vi "Teleop.vi"(10 "Match Info":T1={"Autonomous Elapsed Seconds"=0.0, "TeleOp Elapsed Seconds"=0.0, "Disabled Elapsed Seconds"=0.0, "Visited Autonomous"=FALSE, "Visited TeleOp"=FALSE, "Visited Disabled"=FALSE, "Autonomous Settings"={"Autonomous Style"=enum."Independent", "VI Refnum"=refnum}}, 11 "Call Context":T2) -> ()   [LabVIEW 2013]
doc: "This VI is called for each TeleOp packet received from the DS where the robot is not disabled. It is often used to read from the joysticks and update I/O or to update setpoints for timed control loops. It should complete and return within 20 milliseconds or it may miss DS packets."
uses:
  <vilib>/Rock Robotics/WPI/DriverStation/WPI_DriverStationDerivedRobotMode.ctl
  <vilib>/Rock Robotics/WPI/DriverStation/WPI_DriverStationMatch Info.ctl
  Robot Global Data.vi
  <vilib>/Rock Robotics/WPI/Joystick/WPI_JoystickGetSetRefNum.vi
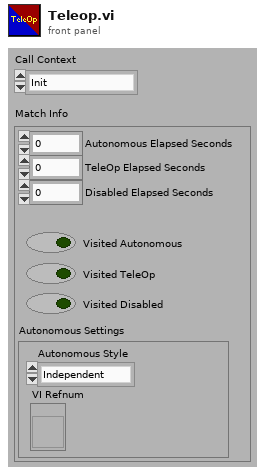
[diagram p1: front panel]
types:
  T1 = typedef "WPI_DriverStationMatch Info.ctl" = cluster{"Autonomous Elapsed Seconds":dbl, "TeleOp Elapsed Seconds":dbl, "Disabled Elapsed Seconds":dbl, "Visited Autonomous":bool, "Visited TeleOp":bool, "Visited Disabled":bool, "Autonomous Settings":cluster{"Autonomous Style":enum16{"Iterative", "Independent"}, "VI Refnum":refnum<vi>}}
  T2 = typedef "WPI_DriverStationDerivedRobotMode.ctl" = enum16{"Init", "Execute", "Stop"}
  T3 = typedef "WPI_JoystickDevRef.ctl" = cluster{"Device":T4}
  T4 = typedef "WPI_JoystickDeviceEnum.ctl" = enum16{"USB 1", "USB 2", "USB 3", "USB 4", "Kinect 1", "Kinect 2"}
  T5 = cluster{"axis 1 (x)":dbl, "axis 2 (y)":dbl, "axis 3 (throttle)":dbl, "axis 4":dbl, "axis 5":dbl, "axis 6":dbl}
  T6 = typedef "WPI_MotorControlDeviceRef.ctl" = cluster{"DeviceStatus":errorcluster, "Type":enum16{"PWM", "CAN"}, "PWM":cluster{"Digital Module":T7, "PWM Channel":T8, "DeadBand":T9}, "CAN":cluster{"Device Number":u8, "Control Mode":T10, "Semaphore":T11, "Max Vout":dbl}, "Invert":bool, "TransformRef":T12, "InvTransformRef":T12}
  T7 = typedef "FPGA_TypedefDigitalModule.ctl" = enum16{"Digital Module 1", "Digital Module 2"}
  T8 = typedef "FPGA_DIOPWMChannel.ctl" = enum8{"PWM 1", "PWM 2", "PWM 3", "PWM 4", "PWM 5", "PWM 6", "PWM 7", "PWM 8", "PWM 9", "PWM 10", "Invalid"}
  T9 = typedef "WPI_PWMDeadband.ctl" = cluster{"Name":string, "maxPositivePwm":i32, "minPositivePwm":i32, "centerPwm":i32, "maxNegativePwm":i32, "minNegativePwm":i32, "angularRange":u16}
  T10 = typedef "WPI_CANJaguar_ControlMode.ctl" = enum8{"Percent VBus", "Current", "Speed", "Position", "Voltage"}
  T11 = typedef "Semaphore RefNum" = refnum<k1>
  T12 = typedef "WPI_PWMTransform_ConPane.ctl" = refnum<vi>
  T13 = typedef "WPI_JoystickButtonState.ctl" = cluster{"Button 1":bool, "Button 2":bool, "Button 3":bool, "Button 4":bool, "Button 5":bool, "Button 6":bool, "Button 7":bool, "Button 8":bool, "Button 9":bool, "Button 10":bool, "Button 11":bool, "Button 12":bool}
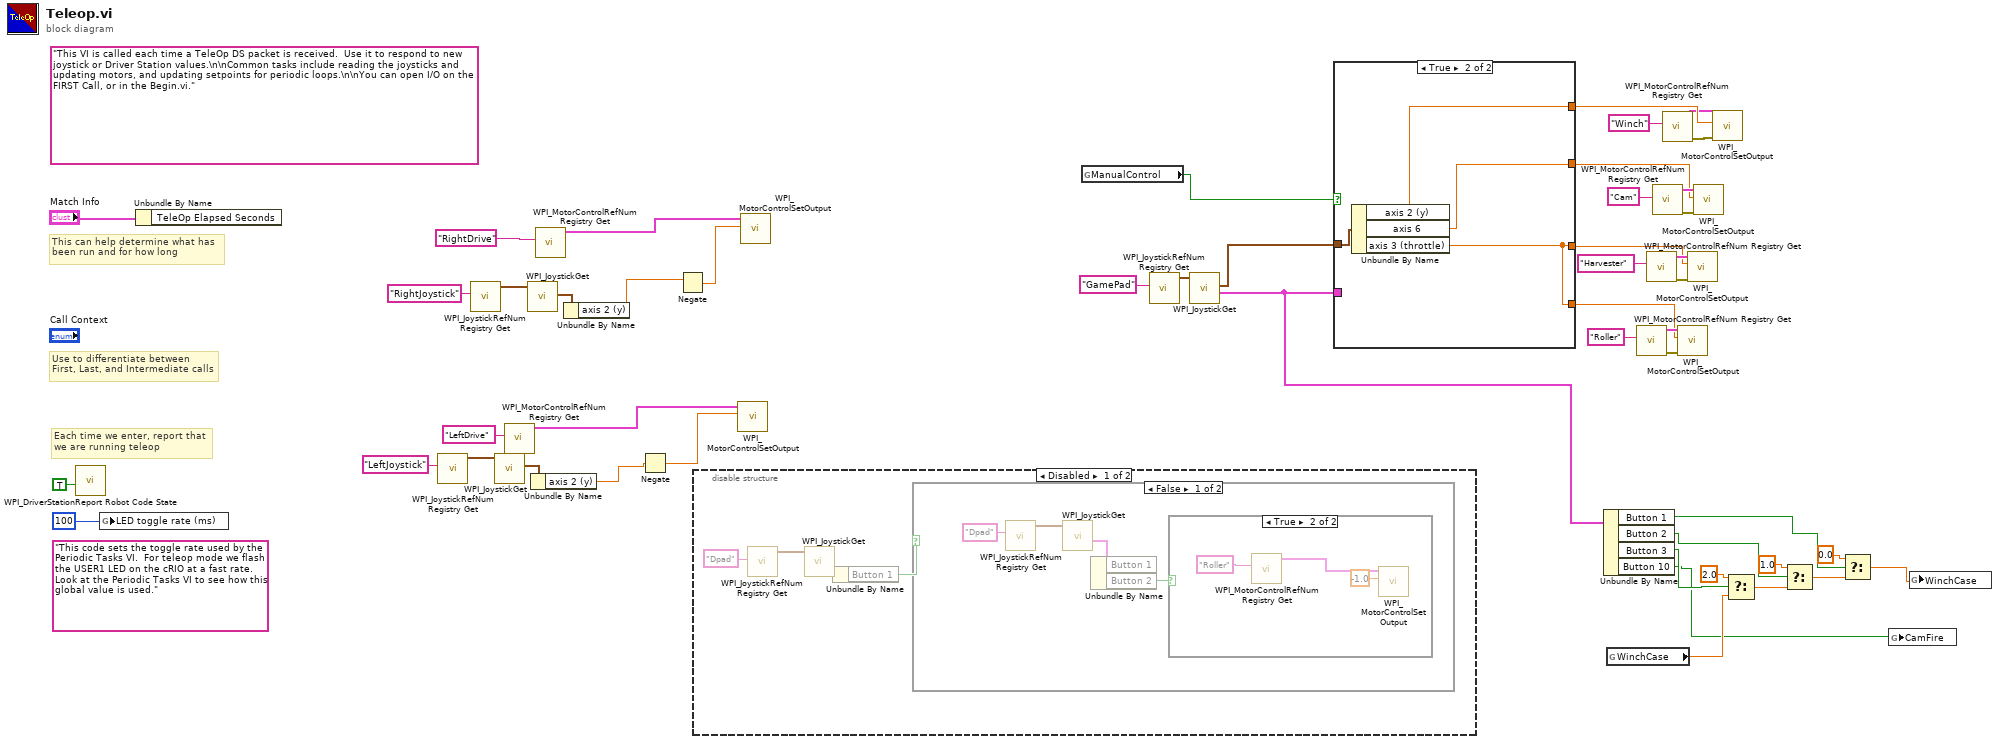
[diagram p0: block diagram]
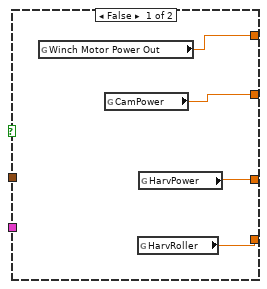
[diagram p2: hidden frame]
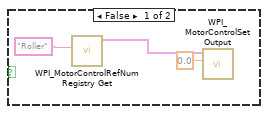
[diagram p3: hidden frame]
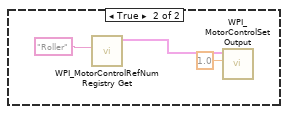
[diagram p4: hidden frame]
diagram:
  (unwired) "This code sets the toggle rate used by the Periodic Tasks VI.  For teleop mode we flash the USER1 LED on the cRIO at a fast rate.  Look at the Periodic Tasks VI to see how this global value is used."
  (unwired) "This VI is called each time a TeleOp DS packet is received.  Use it to respond to new joystick or Driver Station values.\n\nCommon tasks include reading the joysticks and updating motors, and updating setpoints for periodic loops.\n\nYou can open I/O on the FIRST Call, or in the Begin.vi."
  # "Each time we enter, report that\nwe are running teleop"
  # "Use to differentiate between\nFirst, Last, and Intermediate calls"
  # "This can help determine what has\nbeen run and for how long"
  n1 = call <vilib>:"WPI_DriverStationReport Robot Code State.vi"("TeleOp"=TRUE ("Autonomous")) -> ()  [unwired: 10 in, 1 out]
  n2 = global write "Robot Global Data.vi" "LED toggle rate (ms)"(u32 100 ("LED ms toggle rate")) -> ()
  n3 = Unbundle By Name("Match Info") -> ()  [unwired: 1 out]
  n4 = call <vilib>:"WPI_JoystickRefNum Registry Get.vi"("refnum name"="LeftJoystick") -> ("JoystickDevRef"=w38:T3)  [unwired: 9 in, 1 out]
  n5 = call <vilib>:"WPI_JoystickRefNum Registry Get.vi"("refnum name"="RightJoystick") -> ("JoystickDevRef"=w43:T3)  [unwired: 9 in, 1 out]
  n6 = call <vilib>:"WPI_JoystickGet.vi"("JoystickDevRef"=w38) -> ("Axes"=w37:T5)  [unwired: 4 in, 2 out]
  n7 = call <vilib>:"WPI_MotorControlRefNum Registry Get.vi"("refnum name"="LeftDrive") -> ("MotorControlDevRef"=w41:T6)  [unwired: 9 in, 1 out]
  n8 = call <vilib>:"WPI_JoystickGet.vi"("JoystickDevRef"=w43) -> ("Axes"=w42:T5)  [unwired: 4 in, 2 out]
  n9 = Unbundle By Name(w37) -> ("axis 2 (y)"=w36:dbl)
  n10 = call <vilib>:"WPI_MotorControlRefNum Registry Get.vi"("refnum name"="RightDrive") -> ("MotorControlDevRef"=w46:T6)  [unwired: 9 in, 1 out]
  n11 = Unbundle By Name(w42) -> ("axis 2 (y)"=w35:dbl)
  n12 = Negate(x=w36) -> (-x=w34:dbl)
  n13 = Negate(x=w35) -> (-x=w33:dbl)
  n14 = disable-structure shown="Disabled" {
    frame Disabled {
      n15 = call <vilib>:"WPI_JoystickRefNum Registry Get.vi"("refnum name"="Dpad") -> ("JoystickDevRef"=w52:T3)  [unwired: 9 in, 1 out]
      n16 = call <vilib>:"WPI_JoystickGet.vi"("JoystickDevRef"=w52) -> ("Buttons"=w51:T13)  [unwired: 4 in, 2 out]
      n17 = Unbundle By Name(w51) -> ("Button 1"=w50:bool)
      n18 = case shown="False" w50 {
        frame False {
          n19 = call <vilib>:"WPI_JoystickRefNum Registry Get.vi"("refnum name"="Dpad") -> ("JoystickDevRef"=w56:T3)  [unwired: 9 in, 1 out]
          n20 = call <vilib>:"WPI_JoystickGet.vi"("JoystickDevRef"=w56) -> ("Buttons"=w55:T13)  [unwired: 4 in, 2 out]
          n21 = Unbundle By Name(w55) -> ("Button 2"=w54:bool)  [unwired: 1 out]
          n22 = case shown="True" w54 {
            frame False {
              n23 = call <vilib>:"WPI_MotorControlRefNum Registry Get.vi"("refnum name"="Roller") -> ("MotorControlDevRef"=w59:T6)  [unwired: 9 in, 1 out]
              n24 = call <vilib>:"WPI_MotorControlSetOutput.vi"("Output"=0.0, "MotorControlDevRef"=w59) -> ()  [unwired: 7 in, 3 out]
            }
            frame True {
              n25 = call <vilib>:"WPI_MotorControlRefNum Registry Get.vi"("refnum name"="Roller") -> ("MotorControlDevRef"=w62:T6)  [unwired: 9 in, 1 out]
              n26 = call <vilib>:"WPI_MotorControlSetOutput.vi"("Output"=-1.0, "MotorControlDevRef"=w62) -> ()  [unwired: 7 in, 3 out]
            }
          }
        }
        frame True {
          n27 = call <vilib>:"WPI_MotorControlRefNum Registry Get.vi"("refnum name"="Roller") -> ("MotorControlDevRef"=w65:T6)  [unwired: 9 in, 1 out]
          n28 = call <vilib>:"WPI_MotorControlSetOutput.vi"("Output"=1.0, "MotorControlDevRef"=w65) -> ()  [unwired: 7 in, 3 out]
        }
      }
    }
    frame Enabled {
    }
  }
  n29 = call <vilib>:"WPI_MotorControlSetOutput.vi"("Output"=w34, "MotorControlDevRef"=w41) -> ()  [unwired: 7 in, 3 out]
  n30 = call <vilib>:"WPI_MotorControlSetOutput.vi"("Output"=w33, "MotorControlDevRef"=w46) -> ()  [unwired: 7 in, 3 out]
  n31 = global read "Robot Global Data.vi" "ManualControl"() -> (w21:bool)
  n32 = call <vilib>:"WPI_JoystickRefNum Registry Get.vi"("refnum name"="GamePad") -> ("JoystickDevRef"=w31:T3)  [unwired: 9 in, 1 out]
  n33 = call <vilib>:"WPI_JoystickGet.vi"("JoystickDevRef"=w31) -> ("Buttons"=w2:T13, "Axes"=w22:T5)  [unwired: 4 in, 1 out]
  n34 = case shown="True" w21 {
    tunnel: [w70 w71] -> w27
    tunnel: [w69 w71] -> w23
    tunnel: w2 -> [_ _]
    tunnel: w22 -> [_ w74]
    tunnel: [w67 w72] -> w15
    tunnel: [w68 w73] -> w13
    frame False {
      n35 = global read "Robot Global Data.vi" "Winch Motor Power Out"() -> (w67:dbl)
      n36 = global read "Robot Global Data.vi" "CamPower"() -> (w68:dbl)
      n37 = global read "Robot Global Data.vi" "HarvRoller"() -> (w70:dbl)
      n38 = global read "Robot Global Data.vi" "HarvPower"() -> (w69:dbl)
    }
    frame True {
      n39 = Unbundle By Name(w74) -> ("axis 2 (y)"=w72:dbl, "axis 6"=w73:dbl, "axis 3 (throttle)"=w71:dbl)
    }
  }
  n40 = Unbundle By Name(w2) -> ("Button 1"=w5:bool, "Button 2"=w6:bool, "Button 3"=w7:bool, "Button 10"=w1:bool)
  n41 = global read "Robot Global Data.vi" "WinchCase"() -> (w3:dbl)
  n42 = call <vilib>:"WPI_MotorControlRefNum Registry Get.vi"("refnum name"="Roller") -> ("error out"=w28:errorcluster, "MotorControlDevRef"=w29:T6)  [unwired: 9 in]
  n43 = call <vilib>:"WPI_MotorControlRefNum Registry Get.vi"("refnum name"="Harvester") -> ("error out"=w26:errorcluster, "MotorControlDevRef"=w25:T6)  [unwired: 9 in]
  n44 = call <vilib>:"WPI_MotorControlRefNum Registry Get.vi"("refnum name"="Cam") -> ("error out"=w19:errorcluster, "MotorControlDevRef"=w18:T6)  [unwired: 9 in]
  n45 = call <vilib>:"WPI_MotorControlRefNum Registry Get.vi"("refnum name"="Winch") -> ("error out"=w20:errorcluster, "MotorControlDevRef"=w14:T6)  [unwired: 9 in]
  n46 = call <vilib>:"WPI_MotorControlSetOutput.vi"("error in (no error)"=w28, "Output"=w27, "MotorControlDevRef"=w29) -> ()  [unwired: 6 in, 3 out]
  n47 = call <vilib>:"WPI_MotorControlSetOutput.vi"("error in (no error)"=w26, "Output"=w23, "MotorControlDevRef"=w25) -> ()  [unwired: 6 in, 3 out]
  n48 = call <vilib>:"WPI_MotorControlSetOutput.vi"("error in (no error)"=w19, "Output"=w13, "MotorControlDevRef"=w18) -> ()  [unwired: 6 in, 3 out]
  n49 = call <vilib>:"WPI_MotorControlSetOutput.vi"("error in (no error)"=w20, "Output"=w15, "MotorControlDevRef"=w14) -> ()  [unwired: 6 in, 3 out]
  n50 = Select(t=2.0, s=w7, f=w3) -> (s? t:f=w12:dbl)
  n51 = Select(t=1.0, s=w6, f=w12) -> (s? t:f=w11:dbl)
  n52 = Select(t=0.0, s=w5, f=w11) -> (s? t:f=w4:dbl)
  n53 = global write "Robot Global Data.vi" "CamFire"(w1) -> ()
  n54 = global write "Robot Global Data.vi" "WinchCase"(w4) -> ()
